vi "Check Timeout.vi"(8 "error in (no error)":errorcluster, 11 "Helper Loop in":refnum<class "Helper Loop.lvclass">) -> (0 "error out":errorcluster, 2 "timeout":i32, 3 "Helper Loop out":refnum<class "Helper Loop.lvclass">)   [LabVIEW 2024, in "Helper Loop.lvlib" / "Helper Loop.lvclass"]
uses:
  Helper Loop.lvclass
  Helper Loop.lvclass/Helper Loop.ctl
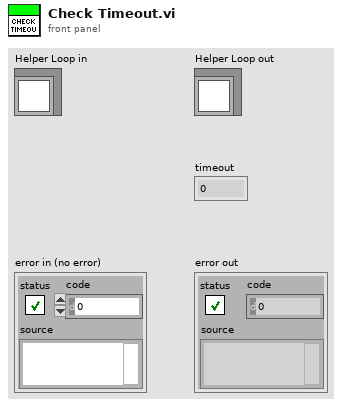
[diagram p1: front panel]
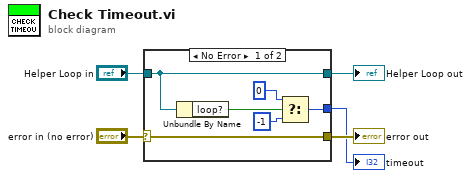
[diagram p0: block diagram]
diagram:
  n1 = case shown="No Error" "error in (no error)" {
    selector: "error in (no error)" -> [w11 w13]
    tunnel: [w11 w13] -> w4
    tunnel: [w10 w12] -> w2
    tunnel: "Helper Loop in" -> [w10 w12]
    tunnel: [w6 _] -> w1
    frame No Error {
      n2 = Unbundle By Name(w10) -> ("loop?"=w9:bool)
      n3 = Select(t=0, s=w9, f=-1) -> (s? t:f=w6:i32)
    }
    frame Error {
    }
  }
  "error out" <- w4
  "Helper Loop out" <- w2
  "timeout" <- w1
